vi "build.vi"(0 "DynamicFrameBuilder in":refnum<class "DynamicFrameBuilder.lvclass">, 5 "WaitForTrigger":bool, 7 "WaitForRxTimeout":u16, 9 "TriggerIRQ":bool, 11 "error in (no error)":errorcluster) -> (4 "DynamicFrameBuilder out":refnum<class "DynamicFrameBuilder.lvclass">, 6 "Frame":T1 {"Data" format="%02x"}, 15 "error out":errorcluster)   [LabVIEW 2016, in "RTModbus.lvlib" / "DynamicFrameBuilder.lvclass"]
uses:
  DynamicFrameBuilder.lvclass
  DataTypes/Frame.ctl
  DynamicFrameBuilder.lvclass/DynamicFrameBuilder.ctl
  RTModbus.lvlib
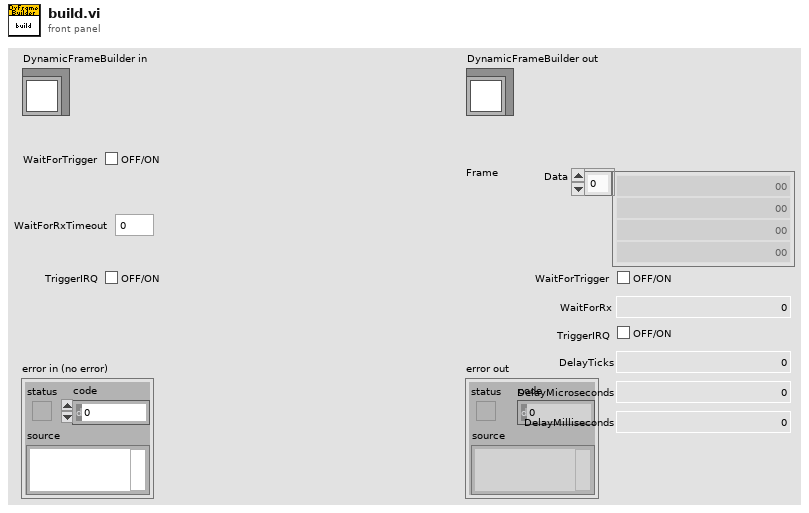
[diagram p1: front panel]
types:
  T1 = typedef "RTModbus.lvlib/Frame.ctl" = cluster{"Data":u8[], "WaitForTrigger":bool, "WaitForRx":u16, "TriggerIRQ":bool, "DelayTicks":u16, "DelayMicroseconds":u16, "DelayMilliseconds":u16}
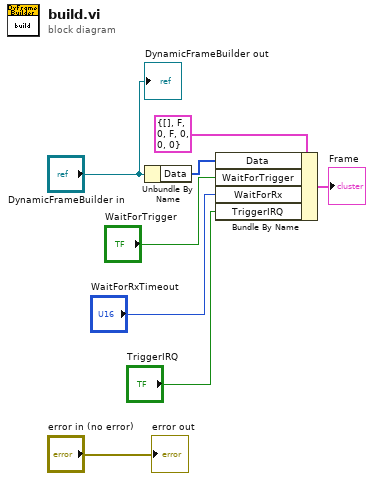
[diagram p0: block diagram]
diagram:
  n1 = Unbundle By Name("DynamicFrameBuilder in") -> ("Data"=w6:u8[])
  n2 = Bundle By Name(cluster=T1 {"Data"=[], "WaitForTrigger"=FALSE, "WaitForRx"=0, "TriggerIRQ"=FALSE, "DelayTicks"=0, "DelayMicroseconds"=0, "DelayMilliseconds"=0} ("Frame"), "Data"=w6, "WaitForTrigger"="WaitForTrigger", "WaitForRx"="WaitForRxTimeout", "TriggerIRQ"="TriggerIRQ") -> (→"Frame":T1)
  "error out" <- "error in (no error)"
  "DynamicFrameBuilder out" <- "DynamicFrameBuilder in"
